vi "Select_data.vi"(7 "condition":string, 8 "error in (no error)":errorcluster caption="错误输入（无错误）", 9 "columns":string[](array[string]), 10 "table":string, 11 "database 输入":refnum<class "database.lvclass">) -> (0 "error out":errorcluster caption="错误输出", 2 "data":string[][](array[string]), 3 "database 输出":refnum<class "database.lvclass">)   [LabVIEW 2016, in "潮位站数据传输.lvlib" / "database.lvclass"]
uses:
  database.lvclass
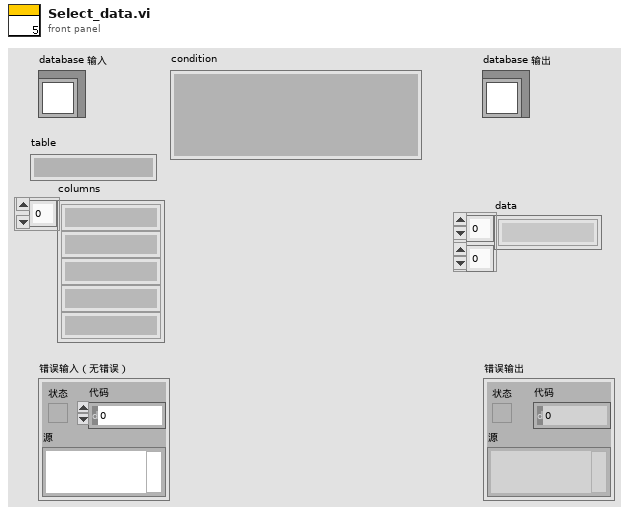
[diagram p1: front panel]
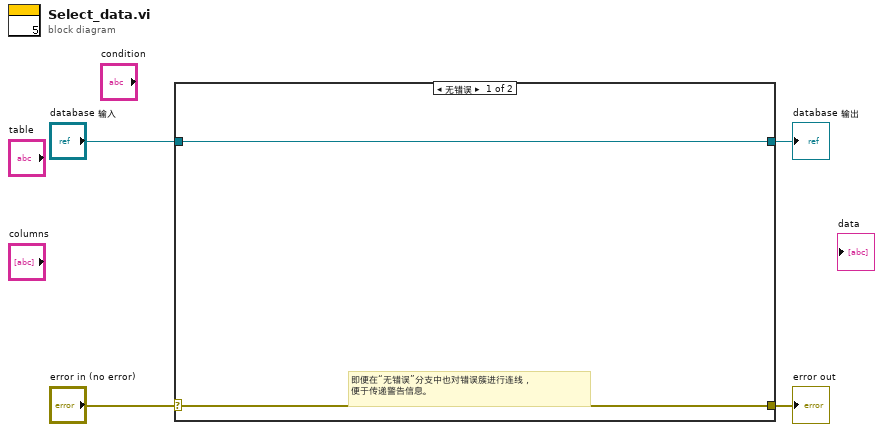
[diagram p0: block diagram]
diagram:
  n1 = case shown="无错误" "error in (no error)" {
    selector: "error in (no error)" -> [w5 w8]
    tunnel: [w5 w8] -> w3
    tunnel: [w6 w7] -> w1
    tunnel: "database 输入" -> [w6 w7]
    frame No Error {
      # "即便在“无错误”分支中也对错误簇进行连线，\n便于传递警告信息。"
    }
    frame Error {
    }
  }
  "error out" <- w3
  "database 输出" <- w1
